vi "firstSuperNodeWhoIs.vi"(6 "Stop Class":string, 8 "error in (no error)":errorcluster, 10 "SuperNode Class":string, 11 "xceNode in":refnum<class "xceNode.lvclass">) -> (0 "error out":errorcluster, 1 "Found":bool, 2 "superNode*":refnum<data-value>, 3 "xceNode out":refnum<class "xceNode.lvclass">)   [LabVIEW 2013, in "xceNode.lvclass"]
doc: "Returns the first superNode who is of type \"SuperNode Class\". The optional input \"Stop Class\" makes it so the search stops if another class is reached first."
uses:
  xceNode.lvclass
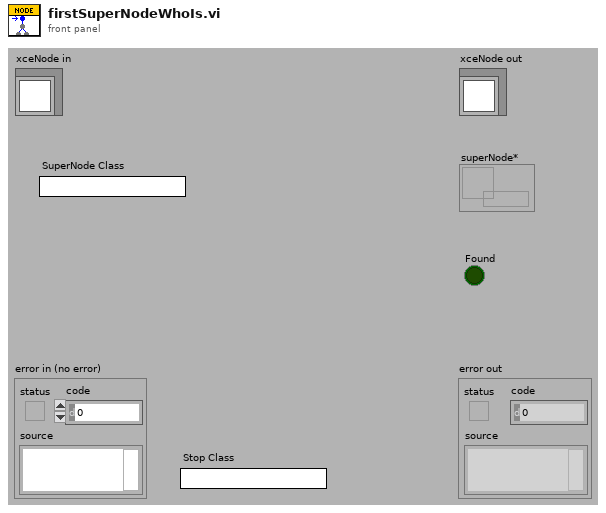
[diagram p1: front panel]
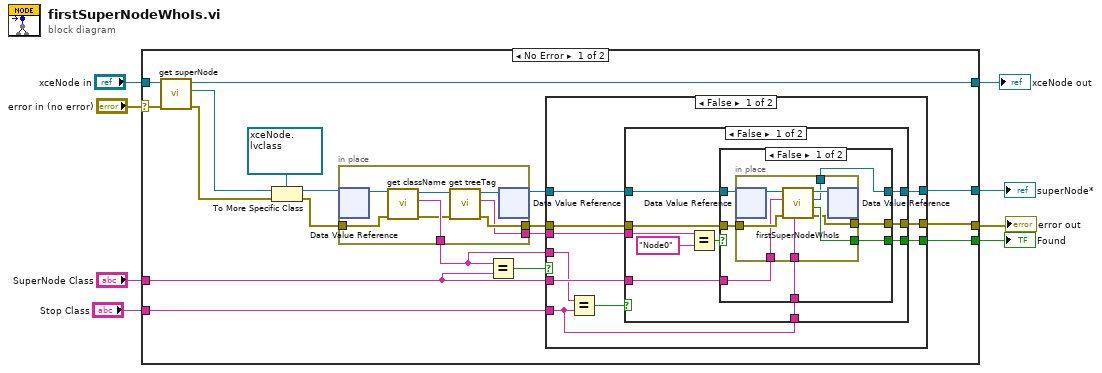
[diagram p0: block diagram]
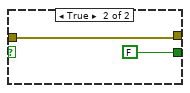
[diagram p2: hidden frame]
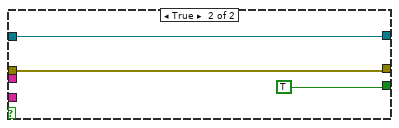
[diagram p4: hidden frame]
diagram:
  n1 = case shown="No Error" "error in (no error)" {
    selector: "error in (no error)" -> [w21 w77]
    tunnel: [w25 w78] -> w6
    tunnel: "xceNode in" -> [w26 w78]
    tunnel: "SuperNode Class" -> [w12 _]
    tunnel: [w16 _] -> w5
    tunnel: [w14 _] -> w4
    tunnel: [w11 w77] -> w3
    tunnel: "Stop Class" -> [w10 _]
    frame No Error {
      n2 = call "get superNode.vi"("error in (no error)"=w21, "xceNode in"=w26) -> ("error out"=w20:errorcluster, "superNode*"=w24:refnum<data-value>, "xceNode out"=w25:refnum<class "xceNode.lvclass">)  [unwired: 7 in]
      n3 = To More Specific Class(target class=refnum<data-value> refnum ("data value reference"), reference=w24, error in=w20) -> (specific class reference=w22:refnum<data-value>, error out=w19:errorcluster)
      n4 = in-place {
        in-place-border: w19 -> [w75]
        in-place-border: [w74] -> w9
        in-place-border: [w70] -> w13
        in-place-border: [w69] -> w15
        n5 = in-place-dvr #1(w22) -> (w76:refnum<class "xceNode.lvclass">)  [unwired: 1 out]
        n6 = call "get className.vi"("error in (no error)"=w75, "xceNode in"=w76) -> ("error out"=w71:errorcluster, "Class name"=w74:string, "xceNode out"=w73:refnum<class "xceNode.lvclass">)  [unwired: 7 in]
        n7 = call "get treeTag.vi"("error in (no error)"=w71, "xceNode in"=w73) -> ("error out"=w70:errorcluster, "treeTag"=w69:string, "xceNode out"=w72:refnum<class "xceNode.lvclass">)  [unwired: 7 in]
        n8 = in-place-dvr #1(w72) -> (w17:refnum<data-value>)  [unwired: 1 out]
      }
      n9 = Equal?(x=w9, y=w12) -> (x = y?=w18:bool)
      n10 = case shown="False" w18 {
        tunnel: w17 -> [w35 w67]
        tunnel: [w34 w67] -> w16
        tunnel: w15 -> [w36 _]
        tunnel: [w33 TRUE] -> w14
        tunnel: w13 -> [w32 w66]
        tunnel: w12 -> [w31 _]
        tunnel: [w30 w66] -> w11
        tunnel: w10 -> [w27 _]
        tunnel: w9 -> [w29 _]
        frame False {
          n11 = Equal?(x=w29, y=w27) -> (x = y?=w28:bool)
          n12 = case shown="False" w28 {
            tunnel: w36 -> [w46 _]
            tunnel: w35 -> [w43 w65]
            tunnel: [w42 w65] -> w34
            tunnel: [w41 _] -> w33
            tunnel: w32 -> [w40 w64]
            tunnel: w31 -> [w39 _]
            tunnel: [w38 w64] -> w30
            tunnel: w27 -> [w37 _]
            frame False {
              n13 = Equal?(x=w46, y="Node0") -> (x = y?=w44:bool)
              n14 = case shown="False" w44 {
                tunnel: w43 -> [w53 _]
                tunnel: [w49 _] -> w42
                tunnel: [w50 FALSE] -> w41
                tunnel: w40 -> [w52 w62]
                tunnel: w39 -> [w51 _]
                tunnel: [w48 w62] -> w38
                tunnel: w37 -> [w47 _]
                frame False {
                  n15 = in-place {
                    in-place-border: w52 -> [w59]
                    in-place-border: w51 -> [w55]
                    in-place-border: [w58] -> w50
                    in-place-border: [w57] -> w49
                    in-place-border: [w56] -> w48
                    in-place-border: w47 -> [w54]
                    n16 = in-place-dvr #2(w53) -> (w61:refnum<class "xceNode.lvclass">)  [unwired: 1 out]
                    n17 = call "firstSuperNodeWhoIs.vi"("Stop Class"=w54, "error in (no error)"=w59, "SuperNode Class"=w55, "xceNode in"=w61) -> ("error out"=w56:errorcluster, "Found"=w58:bool, "superNode*"=w57:refnum<data-value>, "xceNode out"=w60:refnum<class "xceNode.lvclass">)  [unwired: 4 in]
                    n18 = in-place-dvr #2(w60) -> ()  [unwired: 2 out]
                  }
                }
                frame True {
                }
              }
            }
            frame True {
            }
          }
        }
        frame True {
        }
      }
    }
    frame Error {
    }
  }
  "error out" <- w3
  "xceNode out" <- w6
  "superNode*" <- w5
  "Found" <- w4
